vi "MTS_SelectTCSPCBinning.vi"(8 "error in (no error)":errorcluster, 11 "Histograms in":i32[][](array[numeric])=array5x4096[20480 elements]) -> (0 "error out":errorcluster, 1 "TCSPC Binning":i32[][](array[numeric])=[[166, 1512], [1679, 2995]], 2 "Colors":u32[](array[numeric])=[255, 65280, 16711680, 0], 3 "Active":bool[](array[boolean])=[TRUE, TRUE, TRUE, FALSE], 5 "Histogram":i32[][](graph))   [LabVIEW 8.6]
panel:
  in  "L2D2 - Color":u32(colorbox) caption="Color"
  in  "L2D1 - Color":u32(colorbox)=16711680 caption="Color"
  in  "L1D2 - Color":u32(colorbox)=65280 caption="Color"
  in  "L1D1 - Color":u32(colorbox)=255 caption="Color"
  in  "L2D2":bool
  in  "L2D1":bool=TRUE
  in  "L1D2":bool=TRUE
  in  "L1D1":bool=TRUE
  in  "Laser 2":cluster{i32, i32}(slide)={1679, 2995} scale=0.0..3126.0
  in  "Laser 1":cluster{i32, i32}(slide)={166, 1512} scale=0.0..3126.0
  in  "OK Button":bool
  # "Laser 1 - Detector 1"
  # "Laser 1 - Detector 2"
  # "Laser 2 - Detector 1"
  # "Laser 2 - Detector 2"
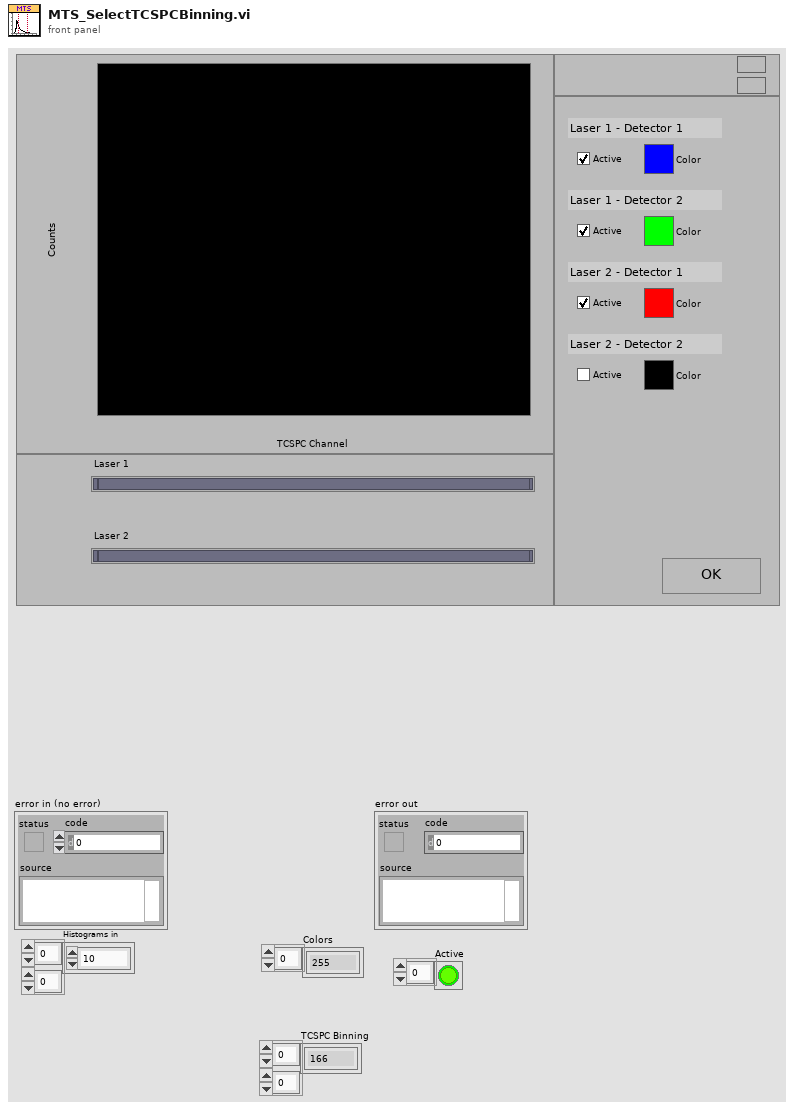
[diagram p1: front panel]
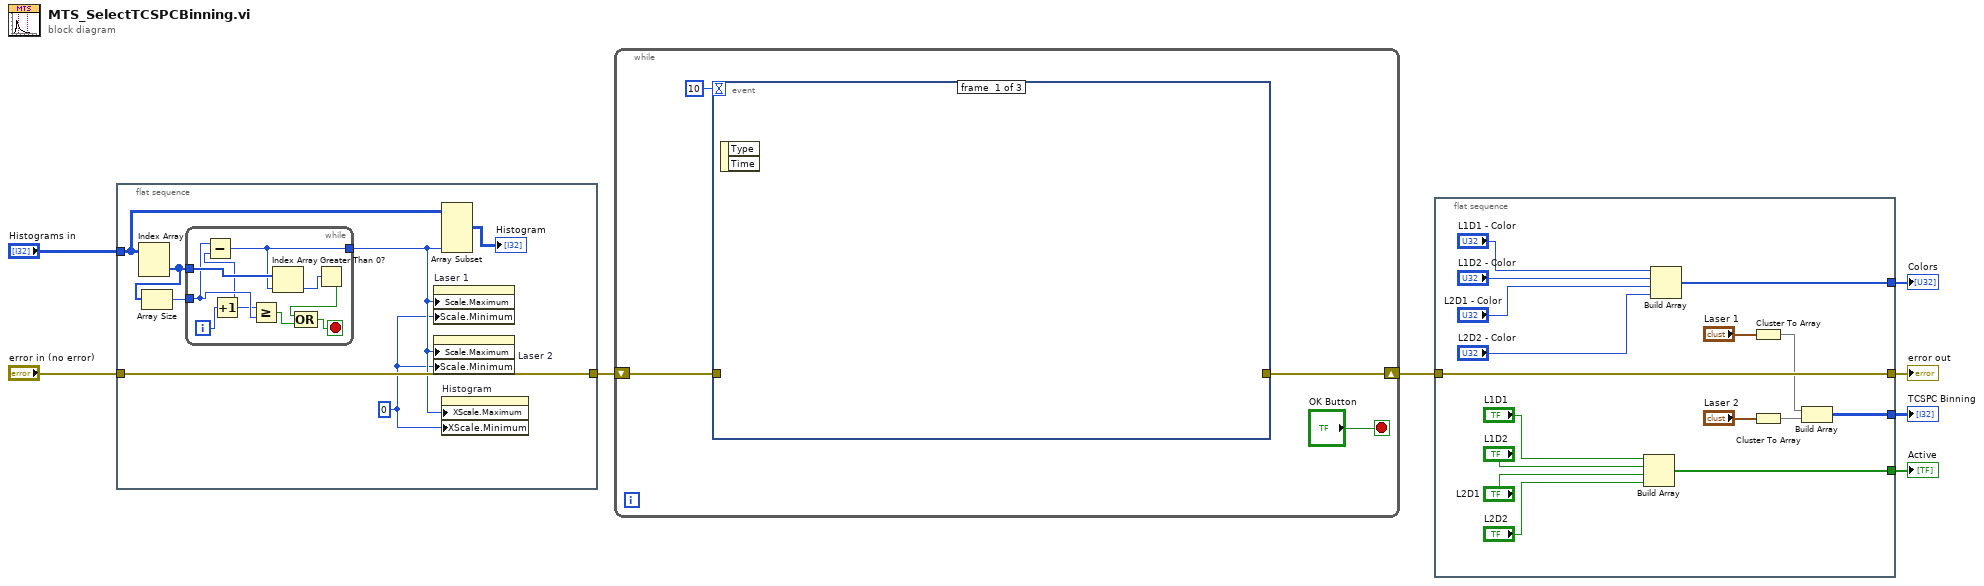
[diagram p0: block diagram]
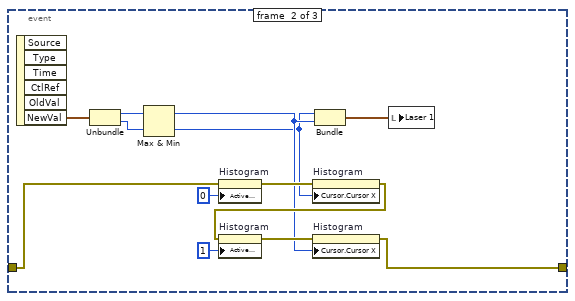
[diagram p2: hidden frame]
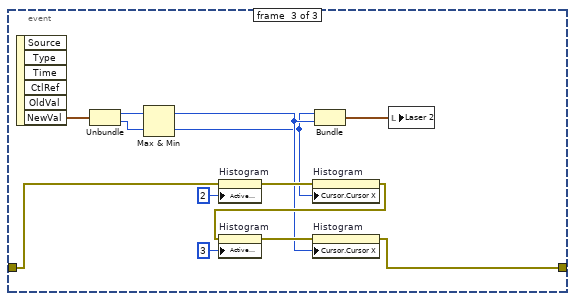
[diagram p3: hidden frame]
diagram:
  n1 = flat-sequence {
    tunnel: "error in (no error)" -> [w13]
    tunnel: [w13] -> w7
    tunnel: "Histograms in" -> [w12]
    frame #0 {
      w9 = 0 ("x-1")
      n2 = Index Array(array=w12) -> (element=w15:i32[])  [unwired: 2 in]
      n3 = Array Size(array=w15) -> (size(s)=w14:i32)
      n4 = while {
        tunnel: w15 -> [w20]
        tunnel: w14 -> [w19]
        tunnel: [w16] -> w10
        i -> [w21]
        stop <- w23 stop-if-true
        n5 = Increment(x=w21) -> (x+1=w18:i32)
        n6 = Subtract(x=w19, y=w18) -> (x-y=w16:i32)
        n7 = Greater Or Equal?(x=w18, y=w19) -> (x >= y?=w24:bool)
        n8 = Index Array(array=w20, index=w16) -> (element=w17:i32)
        n9 = Greater Than 0?(x=w17) -> (x > 0?=w22:bool)
        n10 = Compound Arithmetic op=OR(w22, w24) -> (w23:bool)
      }
      n11 = property on="Laser 1" class="Slide (strict)"("Scale.Maximum"=w10, "Scale.Minimum"=w9) -> ()  [unwired: 2 in, 2 out]
      n12 = property on="Laser 2" class="Slide (strict)"("Scale.Maximum"=w10, "Scale.Minimum"=w9) -> ()  [unwired: 2 in, 2 out]
      n13 = Array Subset(array=w12, length (col)=w10) -> (→"Histogram":i32[][])  [unwired: 3 in]
      n14 = property on="Histogram" class="WFGraph (strict)"("XScale.Maximum"=w10, "XScale.Minimum"=w9) -> ()  [unwired: 2 in, 2 out]
    }
  }
  n15 = while {
    shift-right: [w25] -> w5
    shift-left: w7 -> [w26]
    stop <- "OK Button" stop-if-true
    n16 = event shown="[1] \"Laser 1\": Value Change" {
      selector: _ -> [_ _ _]
      dyn-events: _ -> [_ _ _]
      timeout: 10 -> [_ _ _]
      tunnel: w26 -> [_ w37 w50]
      tunnel: [_ w31 w44] -> w25
      event #0 {
        n17 = event-data() -> ()  [unwired: 3 out]
      }
      event #1 {
        n18 = event-data() -> ("NewVal"=w41:cluster{i32, i32})  [unwired: 6 out]
        n19 = Unbundle(w41) -> (w40:i32, w39:i32)
        n20 = Max & Min(x=w40, y=w39) -> (max(x,y)=w30:i32, min(x,y)=w29:i32)
        n21 = property on="Histogram" class="WFGraph (strict)"(error in=w37, "Active Cursor"=u32 0) -> (error out=w35:errorcluster)  [unwired: 1 in, 1 out]
        n22 = property on="Histogram" class="WFGraph (strict)"(error in=w35, "Cursor.Cursor X"=w29) -> (error out=w32:errorcluster)  [unwired: 1 in, 1 out]
        n23 = property on="Histogram" class="WFGraph (strict)"(error in=w32, "Active Cursor"=u32 1) -> (error out=w33:errorcluster)  [unwired: 1 in, 1 out]
        n24 = property on="Histogram" class="WFGraph (strict)"(error in=w33, "Cursor.Cursor X"=w30) -> (error out=w31:errorcluster)  [unwired: 1 in, 1 out]
        n25 = Bundle(w29, w30) -> (w38:cluster{i32, i32})  [unwired: 1 out]
        n26 = local write "Laser 1"(w38) -> ()
      }
      event #2 {
        n27 = event-data() -> ("NewVal"=w54:cluster{i32, i32})  [unwired: 6 out]
        n28 = Unbundle(w54) -> (w53:i32, w52:i32)
        n29 = Max & Min(x=w53, y=w52) -> (max(x,y)=w43:i32, min(x,y)=w42:i32)
        n30 = property on="Histogram" class="WFGraph (strict)"(error in=w50, "Active Cursor"=u32 2) -> (error out=w48:errorcluster)  [unwired: 1 in, 1 out]
        n31 = property on="Histogram" class="WFGraph (strict)"(error in=w48, "Cursor.Cursor X"=w42) -> (error out=w45:errorcluster)  [unwired: 1 in, 1 out]
        n32 = property on="Histogram" class="WFGraph (strict)"(error in=w45, "Active Cursor"=u32 3) -> (error out=w46:errorcluster)  [unwired: 1 in, 1 out]
        n33 = property on="Histogram" class="WFGraph (strict)"(error in=w46, "Cursor.Cursor X"=w43) -> (error out=w44:errorcluster)  [unwired: 1 in, 1 out]
        n34 = Bundle(w42, w43) -> (w51:cluster{i32, i32})  [unwired: 1 out]
        n35 = local write "Laser 2"(w51) -> ()
      }
    }
  }
  n36 = flat-sequence {
    tunnel: w5 -> [w70]
    tunnel: [w70] -> w4
    tunnel: [w69] -> w2
    tunnel: [w68] -> w3
    tunnel: [w63] -> w1
    frame #0 {
      n37 = Build Array("L1D1", "L1D2", "L2D1", "L2D2") -> (w69:bool[])
      n38 = Build Array("L1D1 - Color", "L1D2 - Color", "L2D1 - Color", "L2D2 - Color") -> (w68:u32[])
      n39 = Cluster To Array(cluster="Laser 1") -> (array=w65:i32[])
      n40 = Cluster To Array(cluster="Laser 2") -> (array=w64:i32[])
      n41 = Build Array(w65, w64) -> (w63:i32[][])
    }
  }
  "error out" <- w4
  "Colors" <- w3
  "Active" <- w2
  "TCSPC Binning" <- w1
